vi "daqio_Tie_File_to_Device.vi"(8 "error in (no error)":errorcluster, 10 "file ID":string, 11 "daq.io type in":T1={"daq.io ref"=refnum, "daq.io API Base"="http://dashboard.daq.io/api/v1", "Device Type Key"="", "Device Key"="", "Account ID"=""}) -> (0 "error out":errorcluster, 3 "daq.io type out":T1={"daq.io ref"=refnum, "daq.io API Base"="http://dashboard.daq.io/api/v1", "Device Type Key"="", "Device Key"="", "Account ID"=""})   [LabVIEW 2013, in "daqio minimal.lvlib"]
doc: "This VI ties a daq.io user file to the current device. This could be a manual or a test report or other useful information that should be used in conjunction with the actual device."
uses:
  daqio minimal.lvlib
  _typedefs/daqio-Type.ctl
  <vilib>/httpClient/ClientHandle.ctl
  _typedefs/daqio-Device.ctl
  <vilib>/Easy HTTP Client/Easy HTTP.lvlib
  <vilib>/httpClient/LabVIEWHTTPClient.lvlib
panel:
  out "Put return":string
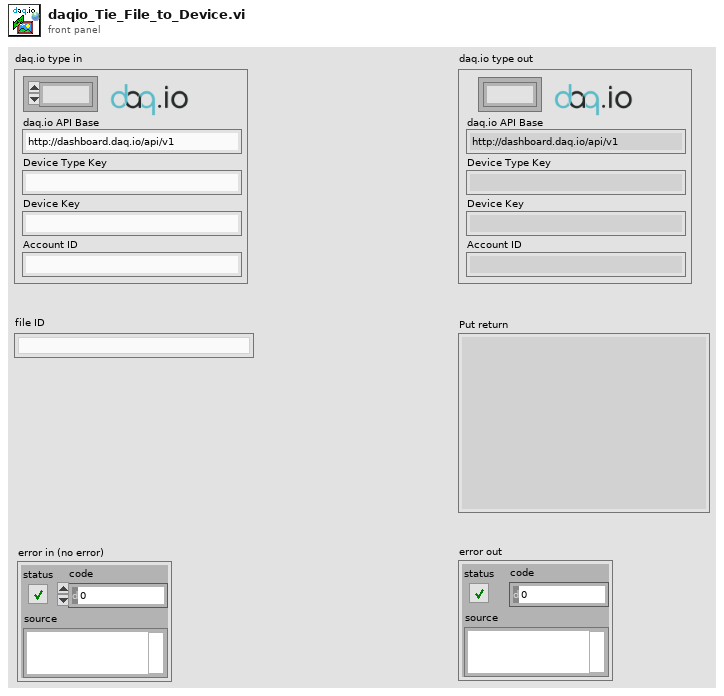
[diagram p1: front panel]
types:
  T1 = typedef "daqio minimal.lvlib/daqio-Type.ctl" = cluster{"daq.io ref":T2, "daq.io API Base":string, "Device Type Key":string, "Device Key":string, "Account ID":string}
  T2 = typedef "LabVIEWHTTPClient.lvlib/ClientHandle.ctl" = refnum<k1>
  T3 = typedef "daqio minimal.lvlib/daqio-Device.ctl" = cluster{"permissions":cluster{"write":string[], "read":string[]}, "id":string, "label":string, "key":string, "device_type_id":string, "tags":cluster{"key":string, "value":string}[], "assets":string[]}
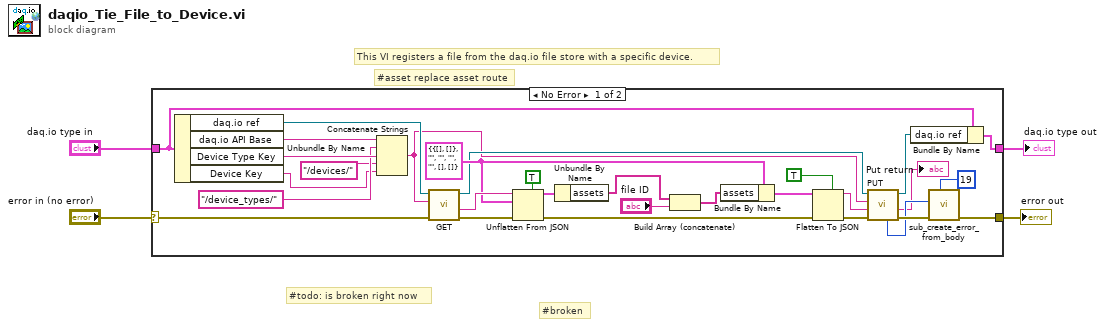
[diagram p0: block diagram]
diagram:
  # "#broken"
  # "#todo: is broken right now"
  # "#asset replace asset route"
  # "This VI registers a file from the daq.io file store with a specific device."
  n1 = case shown="No Error" "error in (no error)" {
    selector: "error in (no error)" -> [w27 w35]
    tunnel: "daq.io type in" -> [w32 w36]
    tunnel: [w31 w36] -> w3
    tunnel: [w34 w35] -> w2
    frame No Error {
      w19 = T3 {"permissions"={"write"=[], "read"=[]}, "id"="", "label"="", "key"="", "device_type_id"="", "tags"=[], "assets"=[]} ("Device")
      n2 = Unbundle By Name(w32) -> ("daq.io ref"=w28:T2, "daq.io API Base"=w33:string, "Device Type Key"=w30:string, "Device Key"=w6:string)
      n3 = Concatenate Strings(w33, "/device_types/", w30, "/devices/" ("string"), w6) -> (w10:string)
      n4 = call <vilib>:"GET.vi"("error in (no error)"=w27, "url"=w10, "client handle"=w28) -> ("error out"=w24:errorcluster, "body"=w25:string, "client handle out"=w11:T2)  [unwired: 4 in, 2 out]
      n5 = Unflatten From JSON(enable LabVIEW extensions? (T)=TRUE, JSON string=w25, type and defaults=w19, error in (no error)=w24) -> (value=w23:T3, error out=w12:errorcluster)  [unwired: 3 in]
      n6 = Unbundle By Name(w23) -> ("assets"=w22:string[])
      n7 = Build Array (concatenate)(w22, "file ID") -> (w20:string[])
      n8 = Bundle By Name(cluster=w19, "assets"=w20) -> (w18:T3)
      n9 = Flatten To JSON(enable LabVIEW extensions? (T)=TRUE, anything=w18, error in (no error)=w12) -> (JSON string=w16:string, 11:w13:errorcluster)
      n10 = call <vilib>:"PUT.vi"("error in (no error)"=w13, "data"=w16, "url"=w10, "client handle"=w11) -> ("error out"=w14:errorcluster, "body"=→"Put return":string, "client handle out"=w15:T2, "HTTP Response Code"=w9:i32)  [unwired: 3 in, 1 out]
      n11 = Bundle By Name(cluster=w32, "daq.io ref"=w15) -> (w31:T1)
      n12 = call "sub_create_error_from_body.vi"("error code"=19, "error in (no error)"=w14, "http code"=w9) -> ("error out"=w34:errorcluster)  [unwired: 8 in]
    }
    frame Error {
    }
  }
  "error out" <- w2
  "daq.io type out" <- w3
